vi "FPGA Init.vi"(8 "error in (no error)":errorcluster, 9 "Device Inputs FIFO":refnum<k33>, 10 "Device Outputs FIFO":refnum<k33>, 11 "Item Ref in":T10 format="%.0x") -> (0 "error out":errorcluster, 3 "RT Data":T1, 4 "FPGA Session Out":refnum<class "FPGA Interface Base.lvclass">)   [LabVIEW 2011, in "Engine Sim RT.lvlib"]
uses:
  Engine Sim RT.lvlib
  <vilib>/NI Veristand/Custom Device API/Custom Device Item Ref.ctl
  <userlib>/_FPGA Interface Advanced Tools/FPGA Interface Base/FPGA Interface Base.lvclass
  TypeDefs/RT Data Cluster.ctl
  Shared/Channel Descriptors.ctl
  Shared/FPGA Write Descriptor.ctl
  Shared/InputChannelTypes.ctl
  <vilib>/rvi/DataTransferAndStorage/Container/Common/niFpgaDataTypeControl.ctl
  Shared/FPGA Read Descriptor.ctl
  Shared/OutputChannelTypes.ctl
  Shared/Status Chan Descriptor.ctl
  Shared/DataReplayVoltageConfig.ctl
  <userlib>/_FPGA Interface Advanced Tools/FPGA Interface Wrapper/TypeDefs/Open Attribute.ctl
  Shared/EngineSimConfig.ctl
  Shared/NTeethConfig.ctl
  Shared/FullyCustomConfig.ctl
  Shared/FullyCustomProfileConfig.ctl
  Shared/FullyCustomCommMode.ctl
  Shared/DataReplayLoopConfig.ctl
  Shared/DataReplayConfig.ctl
  <userlib>/_FPGA Interface Advanced Tools/FPGA Interface Base/FPGA Write By Name - Boolean.vi
  <userlib>/_FPGA Interface Advanced Tools/FPGA Interface Base/FPGA Write By Name - U64.vi
  <vilib>/NI Veristand/Custom Device API/Get Item Property (Boolean).vi
  <vilib>/NI Veristand/Custom Device API/Get Item Property (String).vi
  <vilib>/NI Veristand/Custom Device API/Get Item Property (Variant).vi
  Shared/Engine Simulation Global.vi
  <userlib>/_FPGA Interface Advanced Tools/FPGA Interface Base/Accessors/FPGA Read Session.vi
  <vilib>/NI Veristand/Custom Device API/Custom Device API.lvlib
  Engine Simulation Shared.lvlib
  <userlib>/_FPGA Interface Advanced Tools/FPGA Interface Wrapper/FPGA Interface Wrapper.lvlib
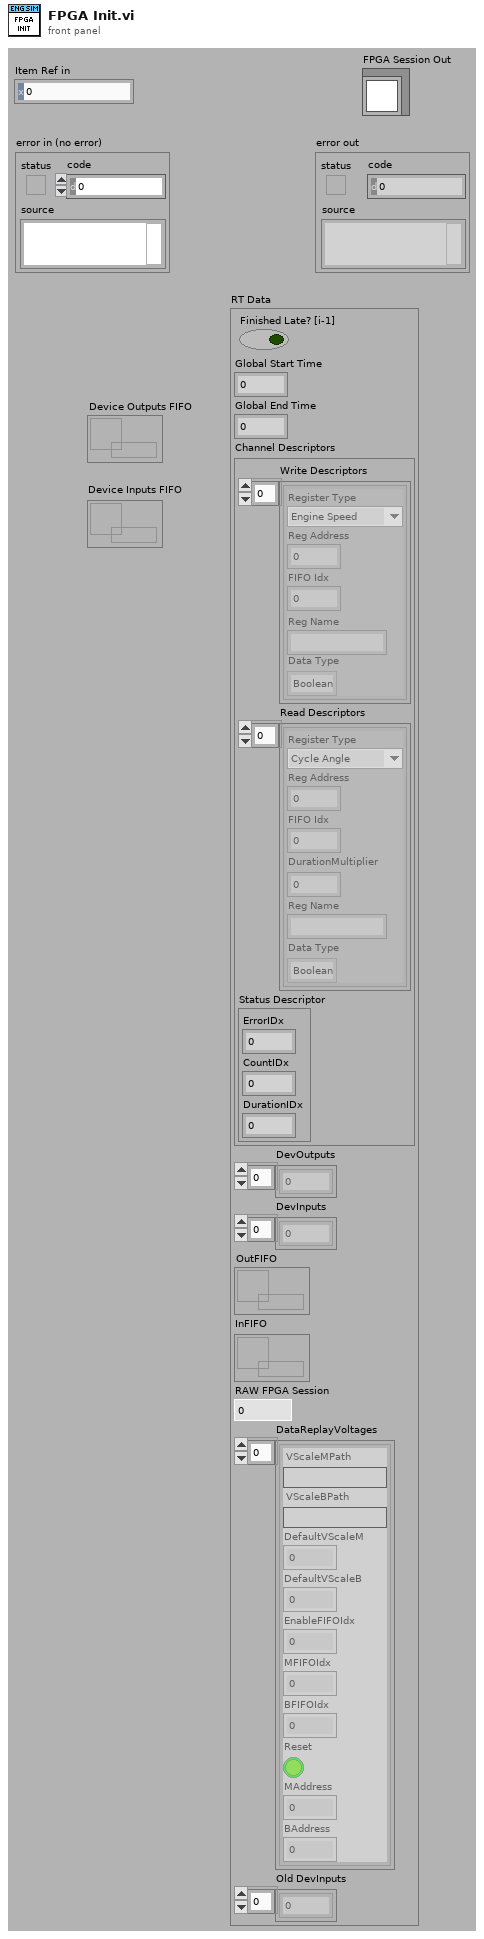
[diagram p1: front panel]
types:
  T1 = typedef "Engine Sim RT.lvlib/RT Data Cluster.ctl" = cluster{"Finished Late? [i-1]":bool, "Global Start Time":i64, "Global End Time":i64, "Channel Descriptors":T2, "DevOutputs":dbl[], "DevInputs":dbl[], "OutFIFO":refnum<k33>, "InFIFO":refnum<k33>, "RAW FPGA Session":u32, "DataReplayVoltages":T9[], "Old DevInputs":dbl[]}
  T2 = typedef "Engine Simulation Shared.lvlib/Channel Descriptors.ctl" = cluster{"Write Descriptors":T3[], "Read Descriptors":T6[], "Status Descriptor":T8}
  T3 = typedef "Engine Simulation Shared.lvlib/FPGA Write Descriptor.ctl" = cluster{"Register Type":T4, "Reg Address":u32, "FIFO Idx":i32, "Reg Name":string, "Data Type":T5}
  T4 = typedef "Engine Simulation Shared.lvlib/InputChannelTypes.ctl" = enum16{"Engine Speed", "Offset"}
  T5 = typedef "niFpgaDataTypeControl.ctl" = enum32{"Boolean", "I8", "I16", "I32", "I64", "U8", "U16", "U32", "U64", "FXP", "CustomControl"}
  T6 = typedef "Engine Simulation Shared.lvlib/FPGA Read Descriptor.ctl" = cluster{"Register Type":T7, "Reg Address":u32, "FIFO Idx":i32, "DurationMultiplier":dbl, "Reg Name":string, "Data Type":T5}
  T7 = typedef "Engine Simulation Shared.lvlib/OutputChannelTypes.ctl" = enum16{"Cycle Angle", "Crank Angle", "Time Duration", "Angle Duration", "Start Angle", "End Angle"}
  T8 = typedef "Engine Simulation Shared.lvlib/Status Chan Descriptor.ctl" = cluster{"ErrorIDx":i32, "CountIDx":i32, "DurationIDx":i32}
  T9 = typedef "Engine Simulation Shared.lvlib/DataReplayVoltageConfig.ctl" = cluster{"VScaleMPath":string, "VScaleBPath":string, "DefaultVScaleM":u32, "DefaultVScaleB":i32, "EnableFIFOIdx":i32, "MFIFOIdx":i32, "BFIFOIdx":i32, "Reset":bool, "MAddress":u32, "BAddress":u32}
  T10 = typedef "Custom Device API.lvlib/Custom Device Item Ref.ctl" = u64
  T11 = typedef "Engine Simulation Shared.lvlib/EngineSimConfig.ctl" = cluster{"NTeeth Configs":T12[], "FullyCustom Configs":T13[], "DataReplayLoops":T16[], "APU.IncrementRate":u64, "DataReplayVoltages":T9[], "Channel Descriptors":T2, "Inputs":i32, "Outputs":i32}
  T12 = typedef "Engine Simulation Shared.lvlib/NTeethConfig.ctl" = cluster{"Base Path":string, "Degrees High Pulse":u64, "Degrees Low Pulse":u64, "TopDeadCenter High?":bool, "Num Teeth Miss":u8, "Missing Teeth Offset":u64, "TDC Offset":u64}
  T13 = typedef "Engine Simulation Shared.lvlib/FullyCustomConfig.ctl" = cluster{"Base Path":string, "Num Profiles":u8, "Num Angles":u8, "Profile Configs":T14[], "Angles FIFO":u64[], "Comm Mode":T15}
  T14 = typedef "Engine Simulation Shared.lvlib/FullyCustomProfileConfig.ctl" = cluster{"Base Path":string, "First Rising?":bool}
  T15 = typedef "Engine Simulation Shared.lvlib/FullyCustomCommMode.ctl" = enum16{"DMA FIFO", "FP Data Transfer"}
  T16 = typedef "Engine Simulation Shared.lvlib/DataReplayLoopConfig.ctl" = cluster{"UpdateRatePath":string, "Loop Tics":u32, "Profile Configs":T17[]}
  T17 = typedef "Engine Simulation Shared.lvlib/DataReplayConfig.ctl" = cluster{"RPMThreshPath":string, "Data":i16[], "VScaleM":u32, "AngleToAdds":u32, "RPMThresh":u64, "NumStr":string, "Number":i8, "AngleToAddsPath":string, "VScaleMPath":string, "VScaleB":i32, "VScaleBPath":string, "CycleAngle?":bool, "CycleAnglePath":string, "ReverseNegate?":bool, "ReverseNegatePath":string}
  T18 = typedef "FPGA Interface Wrapper.lvlib/Open Attribute.ctl" = enum32{"Run (Default)", "No Run"}
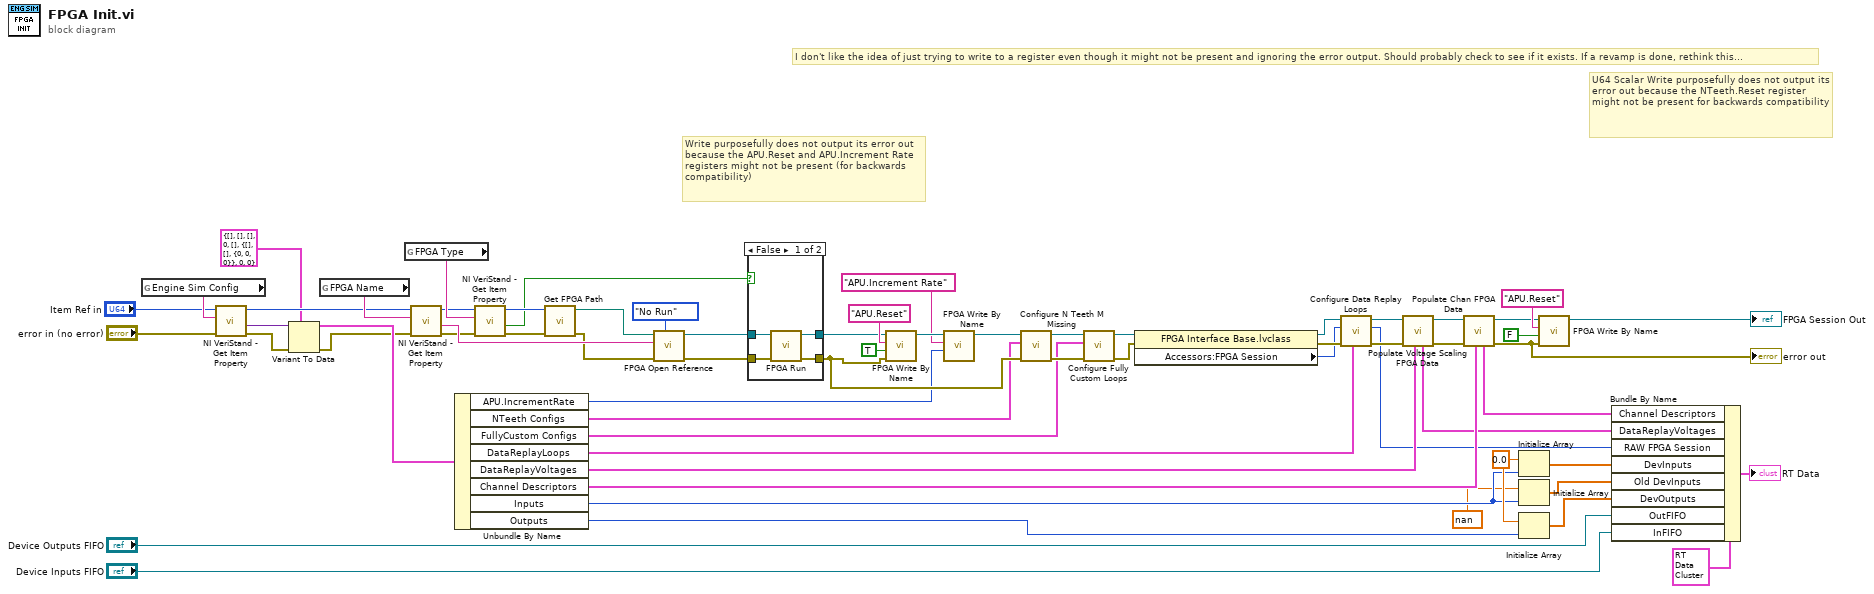
[diagram p0: block diagram]
diagram:
  w4 = 0.0 ("element")
  # "I don't like the idea of just trying to write to a register even though it might not be present and ignoring the error output. Should probably check to see if it exists. If a revamp is done, rethink this..."
  # "U64 Scalar Write purposefully does not output its error out because the NTeeth.Reset register might not be present for backwards compatibility"
  # "Write purposefully does not output its error out because the APU.Reset and APU.Increment Rate registers might not be present (for backwards compatibility)"
  n1 = global read "Engine Simulation Global.vi" "Engine Sim Config"() -> (w60:string)
  n2 = call-poly <vilib>:"NI VeriStand - Get Item Property.vi"("error in (no error)"="error in (no error)", "Property Name"=w60, "Item Ref in"="Item Ref in") -> ("error out"=w23:errorcluster, "Value"=w33:variant, "Item Ref out"=w61:T10)  [unwired: 5 in, 1 out]
  n3 = Variant To Data(error in=w23, type=T11 {"NTeeth Configs"=[], "FullyCustom Configs"=[], "DataReplayLoops"=[], "APU.IncrementRate"=0, "DataReplayVoltages"=[], "Channel Descriptors"={"Write Descriptors"=[], "Read Descriptors"=[], "Status Descriptor"={"ErrorIDx"=0, "CountIDx"=0, "DurationIDx"=0}}, "Inputs"=0, "Outputs"=0} ("Engine Sim Config"), Variant=w33) -> (data=w32:T11, error out=w22:errorcluster)
  n4 = global read "Engine Simulation Global.vi" "FPGA Name"() -> (w62:string)
  n5 = global read "Engine Simulation Global.vi" "FPGA Type"() -> (w56:string)
  n6 = call-poly <vilib>:"NI VeriStand - Get Item Property.vi"("error in (no error)"=w22, "Property Name"=w62, "Item Ref in"=w61) -> ("error out"=w55:errorcluster, "Value"=w65:string, "Item Ref out"=w54:T10)  [unwired: 5 in, 1 out]
  n7 = Unbundle By Name(w32) -> ("APU.IncrementRate"=w27:u64, "NTeeth Configs"=w36:T12[], "FullyCustom Configs"=w35:T13[], "DataReplayLoops"=w31:T16[], "DataReplayVoltages"=w19:T9[], "Channel Descriptors"=w15:T2, "Inputs"=w3:i32, "Outputs"=w9:i32)
  n8 = call-poly <vilib>:"NI VeriStand - Get Item Property.vi"("error in (no error)"=w55, "Property Name"=w56, "Item Ref in"=w54) -> ("error out"=w52:errorcluster, "Value"=w43:bool, "Item Ref out"=w53:T10)  [unwired: 5 in, 1 out]
  n9 = call "Get FPGA Path.vi"("error in (no error)"=w52, "Custom Device Ref"=w53) -> ("error out"=w64:errorcluster, "Path"=w42:path)  [unwired: 8 in]
  n10 = call <userlib>:"FPGA Open Reference.vi"("Run?"=Open_Attribute."No Run", "error in (no error)"=w64, "FPGA Resource"=w65, "Bitfile Path"=w42) -> ("error out"=w47:errorcluster, "FPGA Session"=w46:refnum<class "FPGA Interface Base.lvclass">)  [unwired: 6 in]
  n11 = case shown="False" w43 {
    tunnel: w46 -> [w69 w71]
    tunnel: w47 -> [w68 w70]
    tunnel: [w67 w70] -> w44
    tunnel: [w66 w71] -> w45
    frame False {
      n12 = call <userlib>:"FPGA Run.vi"("error in (no error)"=w68, "FPGA Session In"=w69) -> ("error out"=w67:errorcluster, "FPGA Session Out"=w66:refnum<class "FPGA Interface Base.lvclass">)  [unwired: 8 in]
    }
    frame True {
    }
  }
  n13 = call-poly <userlib>:"FPGA Write By Name.vi"("error in (no error)"=w44, "Value"=TRUE, "Control"="APU.Reset", "FPGA Session In"=w45) -> ("FPGA Session Out"=w30:refnum<class "FPGA Interface Base.lvclass">)  [unwired: 6 in, 1 out]
  n14 = call-poly <userlib>:"FPGA Write By Name.vi"("Value"=w27, "Control"="APU.Increment Rate", "FPGA Session In"=w30) -> ("FPGA Session Out"=w29:refnum<class "FPGA Interface Base.lvclass">)  [unwired: 7 in, 1 out]
  n15 = call "Configure N Teeth M Missing.vi"("error in (no error)"=w44, "NTeeth Configs"=w36, "FPGA Interface Base in"=w29) -> ("error out"=w58:errorcluster, "FPGA Interface Base out"=w59:refnum<class "FPGA Interface Base.lvclass">)  [unwired: 7 in]
  n16 = call "Configure Fully Custom Loops.vi"("error in (no error)"=w58, "FullyCustom Configs"=w35, "FPGA Interface Base in"=w59) -> ("error out"=w40:errorcluster, "FPGA Interface Base out"=w26:refnum<class "FPGA Interface Base.lvclass">)  [unwired: 7 in]
  n17 = property class="FPGA Interface Base.lvclass"(reference=w26, error in=w40) -> (reference out=w37:refnum<class "FPGA Interface Base.lvclass">, error out=w39:errorcluster, "Accessors:FPGA Session"=w38:u32)
  n18 = call "Configure Data Replay Loops.vi"("DataReplayLoops"=w31, "error in (no error)"=w39, "FPGA Session"=w38, "FPGA Interface Base in"=w37) -> ("error out"=w24:errorcluster, "FPGA Session dup"=w12:u32, "FPGA Interface Base out"=w20:refnum<class "FPGA Interface Base.lvclass">)  [unwired: 5 in]
  n19 = call "Populate Voltage Scaling FPGA Data.vi"("DataReplayVoltages in"=w19, "error in (no error)"=w24, "FPGA Interface Base in"=w20) -> ("error out"=w21:errorcluster, "FPGA Interface Base out"=w17:refnum<class "FPGA Interface Base.lvclass">, "DataReplayVoltages out"=w13:T9[])  [unwired: 6 in]
  n20 = call "Populate Chan FPGA Data.vi"("Channel descriptors in"=w15, "error in (no error)"=w21, "FPGA Interface Base in"=w17) -> ("error out"=w18:errorcluster, "FPGA Interface Base out"=w16:refnum<class "FPGA Interface Base.lvclass">, "Channel descriptors out"=w10:T2)  [unwired: 6 in]
  "error out" <- w18
  n21 = Initialize Array(w4, w3) -> (w11:dbl[])
  n22 = Initialize Array(nan ("element"), w3) -> (w1:dbl[])
  n23 = Initialize Array(w4, w9) -> (w8:dbl[])
  n24 = call-poly <userlib>:"FPGA Write By Name.vi"("error in (no error)"=w18, "Value"=FALSE, "Control"="APU.Reset", "FPGA Session In"=w16) -> ("FPGA Session Out"=→"FPGA Session Out":refnum<class "FPGA Interface Base.lvclass">)  [unwired: 6 in, 1 out]
  n25 = Bundle By Name(cluster=T1 {"Finished Late? [i-1]"=FALSE, "Global Start Time"=0, "Global End Time"=0, "Channel Descriptors"={"Write Descriptors"=[], "Read Descriptors"=[], "Status Descriptor"={"ErrorIDx"=0, "CountIDx"=0, "DurationIDx"=0}}, "DevOutputs"=[], "DevInputs"=[], "OutFIFO"=refnum, "InFIFO"=refnum, "RAW FPGA Session"=0, "DataReplayVoltages"=[], "Old DevInputs"=[]} ("Status Information"), "Channel Descriptors"=w10, "DataReplayVoltages"=w13, "RAW FPGA Session"=w12, "DevInputs"=w11, "Old DevInputs"=w1, "DevOutputs"=w8, "OutFIFO"="Device Outputs FIFO", "InFIFO"="Device Inputs FIFO") -> (→"RT Data":T1)
